vi "obj_DataLog Flush List.vi"(5 "entry index in":i32, 6 "tag index in":i32, 7 "method":T1) -> (0 "entries to flush":i32, 1 "entry index out":i32, 2 "tag index out":i32, 3 "unflushed?":bool)   [LabVIEW 2012]
doc: "This object is private to the aggregation buffer. It serves to organize the indices to the per tag oldest unflushed entries in the aggregation buffer, as well as the number of entries to be flushed, into a doubly-linked list. The adding and removing of list nodes as well as looking up the first and last list entries are light weight O(1) operations. These operations are used to allow both FIFO-alike operation (least recently flushed tag first) as well as the flushing of arbitrary tags."
uses:
  typedefs/t_DataLog Flush List Methods.ctl
  subvis/private/glb_DataLog Runtime Parameterisation.vi
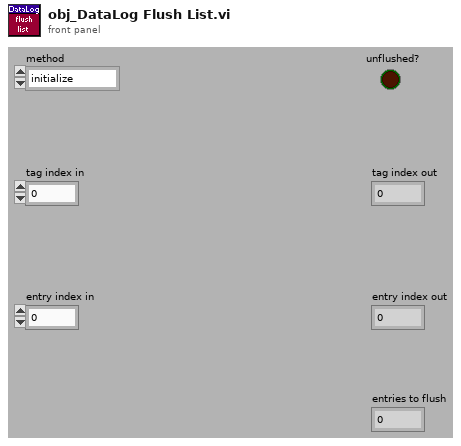
[diagram p1: front panel]
types:
  T1 = typedef "t_DataLog Flush List Methods.ctl" = enum16{"initialize", "add", "remove", "remove next", "info", "info of next", "cleanup"}
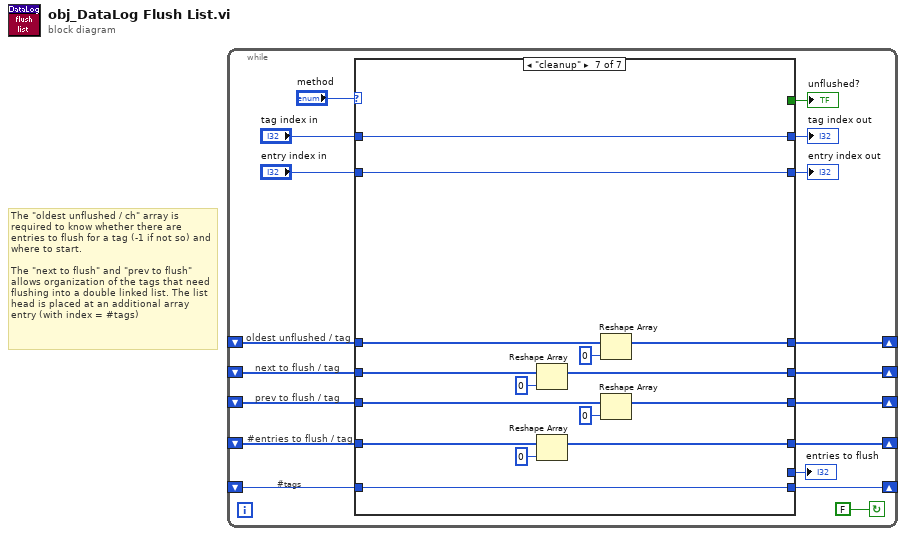
[diagram p0: block diagram]
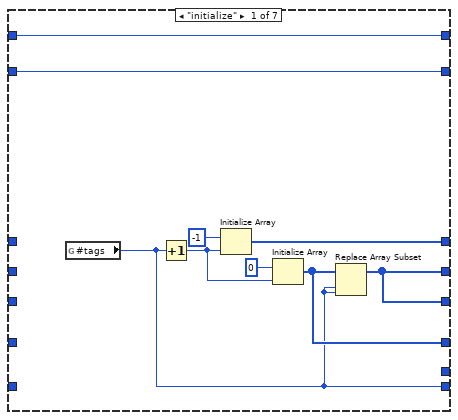
[diagram p2: hidden frame]
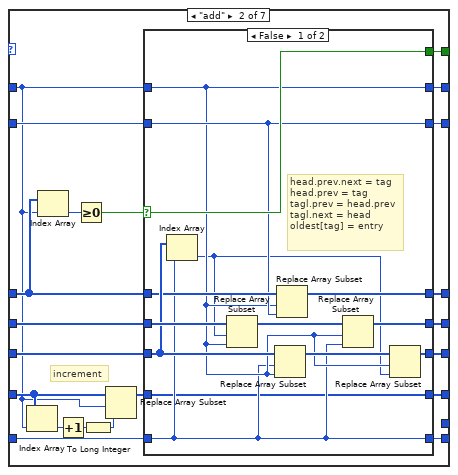
[diagram p3: hidden frame]
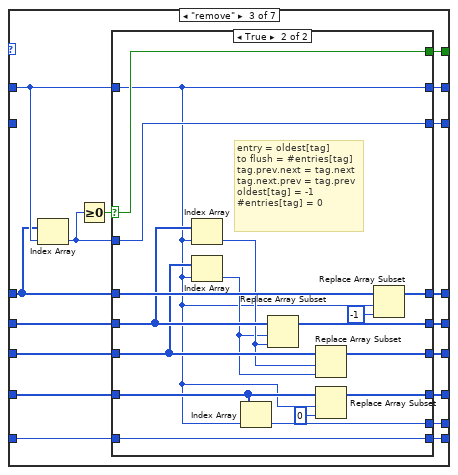
[diagram p5: hidden frame]
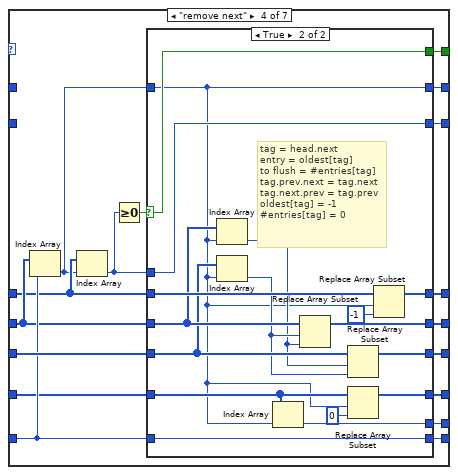
[diagram p7: hidden frame]
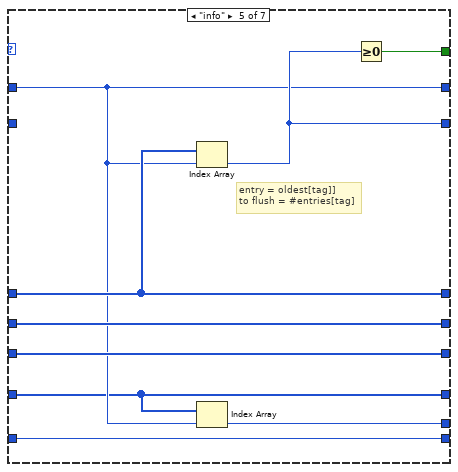
[diagram p9: hidden frame]
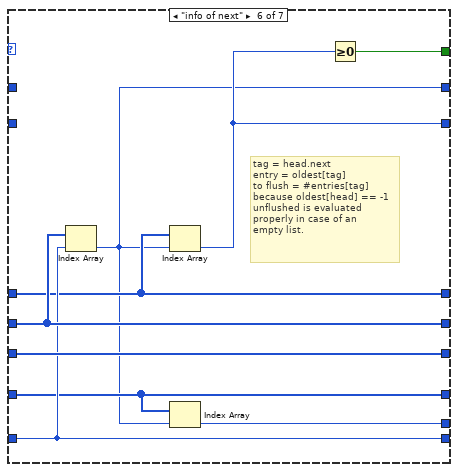
[diagram p10: hidden frame]
diagram:
  # "The \"oldest unflushed / ch\" array is required to know whether there are entries to flush for a tag (-1 if not so) and where to start. \n\nThe \"next to flush\" and \"prev to flush\" allows organization of the tags that need flushing into a double linked list. The list head is placed at an additional array entry (with index = #tags)"
  n1 = while {
    shift-right: [w11] -> _
    shift-left: _ -> [w12]
    shift-right: [w10] -> _
    shift-left: _ -> [w9]
    shift-right: [w7] -> _
    shift-left: _ -> [w8]
    shift-right: [w4] -> _
    shift-left: _ -> [w5]
    shift-right: [w2] -> _
    shift-left: _ -> [w3]
    stop <- FALSE continue-if-true
    # "#entries to flush / tag"
    # "#tags"
    # "prev to flush / tag"
    # "next to flush / tag"
    # "oldest unflushed / tag"
    n2 = case shown="\"cleanup\"" "method" {
      tunnel: [w27 w46 w85 w127 w157 w164 w186] -> w15
      tunnel: "tag index in" -> [w27 w29 w84 _ w157 _ w186]
      tunnel: "entry index in" -> [w26 w44 _ _ _ _ w187]
      tunnel: [w26 w45 w83 w126 w158 w169 w187] -> w13
      tunnel: w12 -> [_ w38 w76 w118 w160 w166 w184]
      tunnel: [w25 w39 w77 w122 w160 w166 w173] -> w11
      tunnel: w9 -> [_ w43 w82 w119 w163 w171 w177]
      tunnel: [w22 w42 w81 w125 w163 w171 w174] -> w10
      tunnel: w8 -> [_ w40 w79 w123 w162 w172 w179]
      tunnel: [w22 w41 w80 w124 w162 w172 w175] -> w7
      tunnel: [_ w47 w86 w128 w159 w170 _] -> w6
      tunnel: w5 -> [_ w37 w75 w120 w161 w168 w185]
      tunnel: [w19 w36 w74 w121 w161 w168 w185] -> w4
      tunnel: w3 -> [_ w32 w72 w115 w156 w165 w178]
      tunnel: [w20 w34 w71 w114 w156 w165 w176] -> w2
      tunnel: [_ _ w73 w113 w155 w167 _] -> w1
      frame "initialize" {
        n3 = global read "glb_DataLog Runtime Parameterisation.vi" "#tags"() -> (w19:i32)
        n4 = Increment(x=w19) -> (x+1=w21:i32)
        n5 = Initialize Array(-1, w21) -> (w25:i32[])
        n6 = Initialize Array(0, w21) -> (w20:i32[])
        n7 = Replace Array Subset(array=w20, new element=w19, index=w19) -> (w22:i32[])
      }
      frame "add" {
        # "increment"
        n8 = Index Array(array=w32, index=w29) -> (element=w33:i32)
        n9 = Index Array(array=w38, index=w29) -> (element=w35:i32)
        n10 = Increment(x=w33) -> (x+1=w30:i32)
        n11 = Greater Or Equal To 0?(x=w35) -> (x >= 0?=w48:bool)
        n12 = To Long Integer(number=w30) -> (32bit integer=w28:i32)
        n13 = Replace Array Subset(array=w32, new element=w28, index=w29) -> (w31:i32[])
        n14 = case shown="False" w48 {
          selector: w48 -> [w62 w70]
          tunnel: [w62 w70] -> w47
          tunnel: w29 -> [w52 w69]
          tunnel: [w52 w69] -> w46
          tunnel: w44 -> [w57 w68]
          tunnel: [w57 w68] -> w45
          tunnel: w43 -> [w61 w67]
          tunnel: [w55 w67] -> w42
          tunnel: [w54 w66] -> w41
          tunnel: w40 -> [w60 w66]
          tunnel: [w58 w64] -> w39
          tunnel: w38 -> [w59 w64]
          tunnel: w37 -> [w51 w65]
          tunnel: [w51 w65] -> w36
          tunnel: w31 -> [w49 w63]
          tunnel: [w49 w63] -> w34
          frame False {
            # "head.prev.next = tag\nhead.prev = tag\ntagl.prev = head.prev\ntagl.next = head\noldest[tag] = entry"
            n15 = Index Array(array=w60, index=w51) -> (element=w50:i32)
            n16 = Replace Array Subset(array=w61, new element=w52, index=w50) -> (w56:i32[])
            n17 = Replace Array Subset(array=w60, new element=w52, index=w51) -> (w53:i32[])
            n18 = Replace Array Subset(array=w59, new element=w57, index=w52) -> (w58:i32[])
            n19 = Replace Array Subset(array=w56, new element=w51, index=w52) -> (w55:i32[])
            n20 = Replace Array Subset(array=w53, new element=w50, index=w52) -> (w54:i32[])
          }
          frame True {
          }
        }
      }
      frame "remove" {
        n21 = Index Array(array=w76, index=w84) -> (element=w78:i32)
        n22 = Greater Or Equal To 0?(x=w78) -> (x >= 0?=w87:bool)
        n23 = case shown="True" w87 {
          selector: w87 -> [w95 w112]
          tunnel: [w95 w112] -> w86
          tunnel: w84 -> [w94 w96]
          tunnel: [w94 w96] -> w85
          tunnel: [w89 w103] -> w83
          tunnel: w82 -> [w93 w106]
          tunnel: [w93 w111] -> w81
          tunnel: [w92 w110] -> w80
          tunnel: w79 -> [w92 w105]
          tunnel: w78 -> [w89 w103]
          tunnel: [w90 w108] -> w77
          tunnel: w76 -> [w90 w109]
          tunnel: w75 -> [w91 w104]
          tunnel: [w91 w104] -> w74
          tunnel: [_ w99] -> w73
          tunnel: w72 -> [w88 w98]
          tunnel: [w88 w97] -> w71
          frame False {
          }
          frame True {
            # "entry = oldest[tag]\nto flush = #entries[tag]\ntag.prev.next = tag.next\ntag.next.prev = tag.prev\noldest[tag] = -1\n#entries[tag] = 0"
            n24 = Index Array(array=w106, index=w96) -> (element=w102:i32)
            n25 = Index Array(array=w105, index=w96) -> (element=w101:i32)
            n26 = Index Array(array=w98, index=w96) -> (element=w99:i32)
            n27 = Replace Array Subset(array=w106, new element=w102, index=w101) -> (w111:i32[])
            n28 = Replace Array Subset(array=w105, new element=w101, index=w102) -> (w110:i32[])
            n29 = Replace Array Subset(array=w98, new element=0 ("new element/subarray"), index=w96) -> (w97:i32[])
            n30 = Replace Array Subset(array=w109, new element=-1 ("new element/subarray"), index=w96) -> (w108:i32[])
          }
        }
      }
      frame "remove next" {
        n31 = Index Array(array=w119, index=w120) -> (element=w116:i32)
        n32 = Index Array(array=w118, index=w116) -> (element=w117:i32)
        n33 = Greater Or Equal To 0?(x=w117) -> (x >= 0?=w129:bool)
        n34 = case shown="True" w129 {
          selector: w129 -> [w137 w154]
          tunnel: [w137 w154] -> w128
          tunnel: w116 -> [w136 w138]
          tunnel: [w136 w138] -> w127
          tunnel: [w131 w145] -> w126
          tunnel: w119 -> [w135 w148]
          tunnel: [w135 w153] -> w125
          tunnel: [w134 w152] -> w124
          tunnel: w123 -> [w134 w147]
          tunnel: w117 -> [w131 w145]
          tunnel: [w132 w150] -> w122
          tunnel: w118 -> [w132 w151]
          tunnel: w120 -> [w133 w146]
          tunnel: [w133 w146] -> w121
          tunnel: w115 -> [w130 w142]
          tunnel: [w130 w141] -> w114
          tunnel: [_ w139] -> w113
          frame False {
          }
          frame True {
            # "tag = head.next\nentry = oldest[tag]\nto flush = #entries[tag]\ntag.prev.next = tag.next\ntag.next.prev = tag.prev\noldest[tag] = -1\n#entries[tag] = 0"
            n35 = Index Array(array=w148, index=w138) -> (element=w143:i32)
            n36 = Index Array(array=w147, index=w138) -> (element=w144:i32)
            n37 = Index Array(array=w142, index=w138) -> (element=w139:i32)
            n38 = Replace Array Subset(array=w148, new element=w143, index=w144) -> (w153:i32[])
            n39 = Replace Array Subset(array=w147, new element=w144, index=w143) -> (w152:i32[])
            n40 = Replace Array Subset(array=w142, new element=0 ("new element/subarray"), index=w138) -> (w141:i32[])
            n41 = Replace Array Subset(array=w151, new element=-1 ("new element/subarray"), index=w138) -> (w150:i32[])
          }
        }
      }
      frame "info" {
        # "entry = oldest[tag]]\nto flush = #entries[tag]"
        n42 = Index Array(array=w160, index=w157) -> (element=w158:i32)
        n43 = Index Array(array=w156, index=w157) -> (element=w155:i32)
        n44 = Greater Or Equal To 0?(x=w158) -> (x >= 0?=w159:bool)
      }
      frame "info of next" {
        # "tag = head.next\nentry = oldest[tag]\nto flush = #entries[tag]\nbecause oldest[head] == -1\nunflushed is evaluated\nproperly in case of an\nempty list."
        n45 = Index Array(array=w171, index=w168) -> (element=w164:i32)
        n46 = Index Array(array=w166, index=w164) -> (element=w169:i32)
        n47 = Index Array(array=w165, index=w164) -> (element=w167:i32)
        n48 = Greater Or Equal To 0?(x=w169) -> (x >= 0?=w170:bool)
      }
      frame "cleanup" {
        n49 = Reshape Array(w177, 0 ("dimension size")) -> (w174:i32[])
        n50 = Reshape Array(w178, 0 ("dimension size")) -> (w176:i32[])
        n51 = Reshape Array(w184, 0 ("dimension size")) -> (w173:i32[])
        n52 = Reshape Array(w179, 0 ("dimension size")) -> (w175:i32[])
      }
    }
    "unflushed?" <- w6
    "entry index out" <- w13
    "tag index out" <- w15
    "entries to flush" <- w1
  }
